vi "FGV_Bool_Array.vi"(8 "Array In":bool[](array[boolean]), 11 "Enum":enum16{"read", "write"}(ring)) -> (3 "Array Out":bool[](array[boolean]))   [LabVIEW 2020]
panel:
  out "error out":errorcluster
  in  "error in":errorcluster
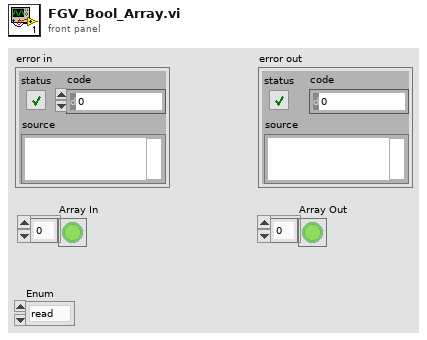
[diagram p1: front panel]
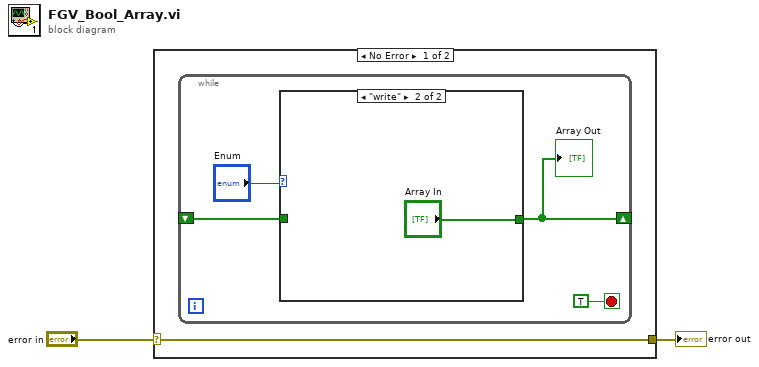
[diagram p0: block diagram]
diagram:
  n1 = case shown="No Error" "error in" {
    selector: "error in" -> [w3 w10]
    tunnel: [w3 w10] -> w1
    frame No Error {
      n2 = while {
        shift-right: [w4] -> _
        shift-left: _ -> [w5]
        stop <- TRUE stop-if-true
        n3 = case shown="\"write\"" "Enum" {
          tunnel: [w8 "Array In"] -> w4
          tunnel: w5 -> [w8 _]
          frame "read", Default {
          }
          frame "write" {
          }
        }
        "Array Out" <- w4
      }
    }
    frame Error {
    }
  }
  "error out" <- w1
